vi "2023_day07_Task2(subVI Best Combination with Joker).vi"(9 "Number of Jokers":i32, 10 "Data In":i32[](array[numeric])) -> (2 "Data Out":i32[](array[numeric]))   [LabVIEW 2021]
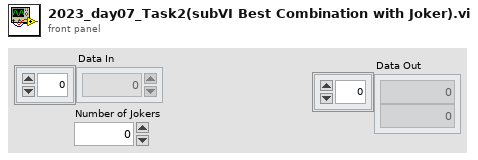
[diagram p1: front panel]
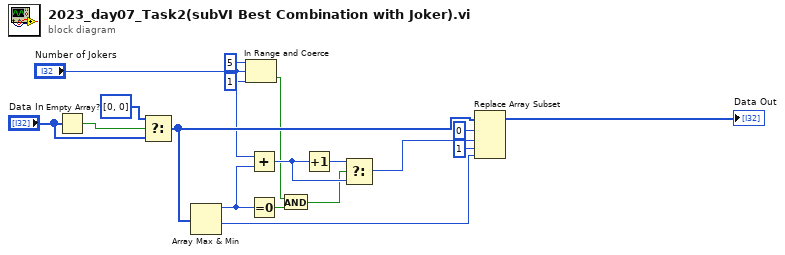
[diagram p0: block diagram]
diagram:
  n1 = Empty Array?(array="Data In") -> (empty?=w14:bool)
  n2 = Select(t=i32[] [0, 0], s=w14, f="Data In") -> (s? t:f=w12:i32[])
  n3 = Array Max & Min(array=w12) -> (max value=w7:i32, min value=w17:i32)  [unwired: 2 out]
  n4 = In Range and Coerce(upper limit=5, x="Number of Jokers", lower limit=1) -> (In Range?=w3:bool)  [unwired: 1 out]
  n5 = Add(x="Number of Jokers", y=w7) -> (x+y=w8:i32)
  n6 = Equal To 0?(x=w7) -> (x = 0?=w6:bool)
  n7 = And(x=w3, y=w6) -> (x .and. y?=w5:bool)
  n8 = Increment(x=w8) -> (x+1=w10:i32)
  n9 = Select(t=w10, s=w5, f=w8) -> (s? t:f=w9:i32)
  n10 = Replace Array Subset(array=w12, new element #1=w9, index #1=0 ("index"), new element #2=w17, index #2=1 ("index")) -> (→"Data Out":i32[])
